vi "Write Lockin Digitizer Driver.vi"(8 "error in (no error)":errorcluster, 10 "Lockin Digitizer Driver.lvclass":refnum<class "Lockin Digitizer Driver.lvclass">, 11 "Lockin Digitizer in":refnum<class "Lockin Digitizer.lvclass">) -> (0 "error out":errorcluster, 3 "Lockin Digitizer out":refnum<class "Lockin Digitizer.lvclass">)   [LabVIEW 2021, in "Lockin Digitizer.lvclass"]
uses:
  Lockin Digitizer.lvclass
  Lockin Digitizer.lvclass/Lockin Digitizer.ctl
  NHMFL_Core/Libraries/Instruments/Pulse Driver/Lockin Digitizer Driver/Lockin Digitizer Driver.lvclass
  C:/GitHub/NHMFL_Core/Libraries/Instruments/Pulse Driver/Pulse Driver.lvclass
  C:/GitHub/NHMFL_Core/Libraries/Instruments/Instrument Driver/Instrument Driver.lvclass
  C:/GitHub/NHMFL_Core/Libraries/Instruments/Pulse Driver/Lockin Digitizer Driver/Lockin Digitizer Driver.lvclass
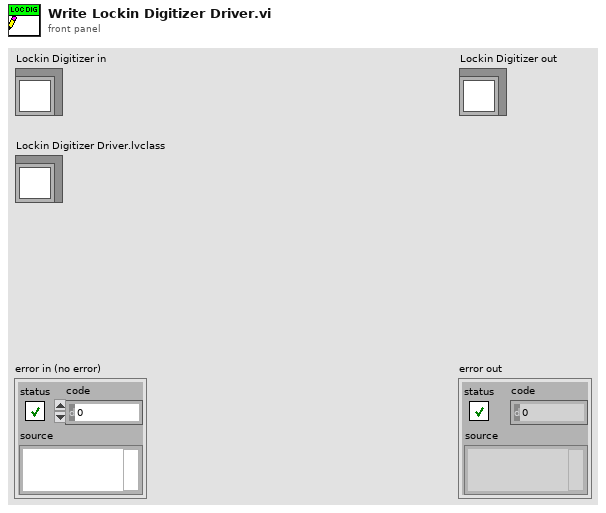
[diagram p1: front panel]
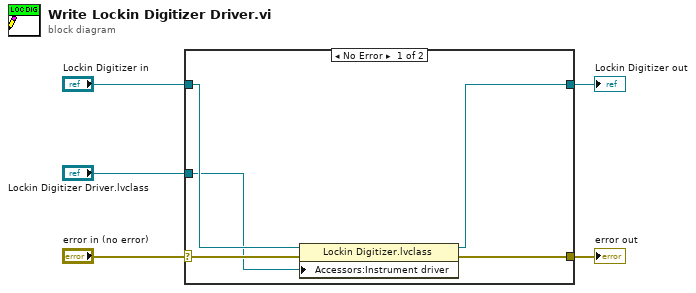
[diagram p0: block diagram]
diagram:
  n1 = case shown="No Error" "error in (no error)" {
    selector: "error in (no error)" -> [w10 w11]
    tunnel: [w9 w11] -> w4
    tunnel: [w7 w12] -> w2
    tunnel: "Lockin Digitizer in" -> [w8 w12]
    tunnel: "Lockin Digitizer Driver.lvclass" -> [w6 _]
    frame No Error {
      n2 = property class="Lockin Digitizer.lvclass"(reference=w8, error in=w10, "Accessors:Instrument driver"=w6) -> (reference out=w7:refnum<class "Lockin Digitizer.lvclass">, error out=w9:errorcluster)
    }
    frame Error {
    }
  }
  "error out" <- w4
  "Lockin Digitizer out" <- w2
